vi "Spy Flush and Check for Specific Call.vi"(8 "error in (no error)":errorcluster, 10 "Specific Call":string, 11 "Mock Rig Process In":refnum<class "Mock Process.lvclass">) -> (0 "error out":errorcluster, 2 "Occured?":bool, 3 "Mock Rig Process Out":refnum<class "Mock Process.lvclass">)   [LabVIEW 2020, in "Mock Process.lvclass"]
uses:
  Mock Process.lvclass
  Mock Process.lvclass/Mock Process.ctl
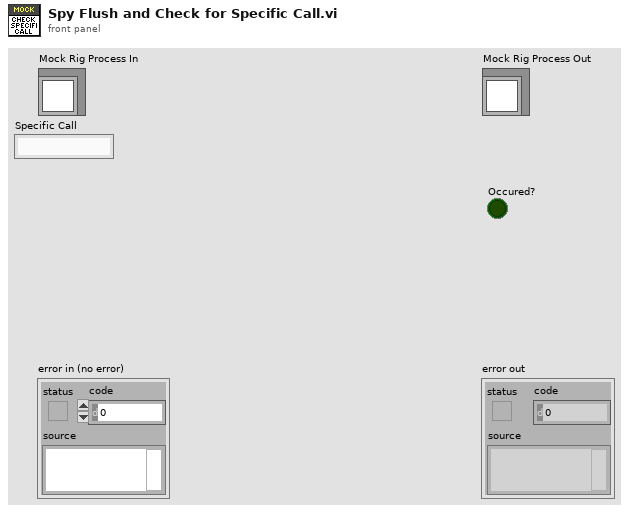
[diagram p1: front panel]
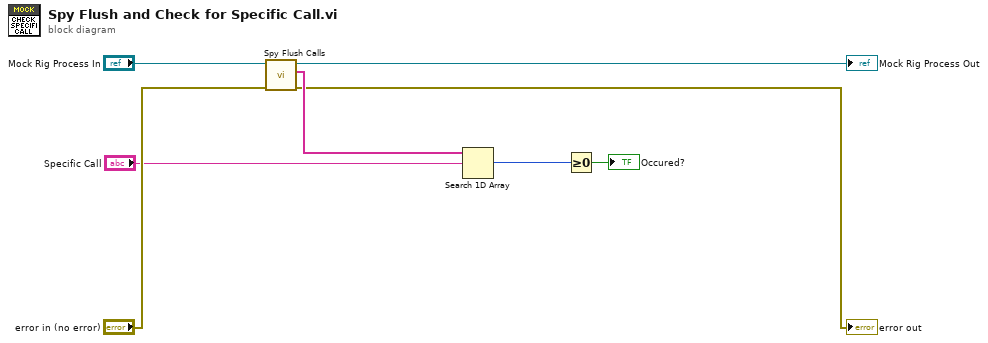
[diagram p0: block diagram]
diagram:
  n1 = call "Spy Flush Calls.vi"("error in (no error)"="error in (no error)", "Mock Process In"="Mock Rig Process In") -> ("error out"=→"error out":errorcluster, "Message"=w5:string[], "Mock Process Out"=→"Mock Rig Process Out":refnum<class "Mock Process.lvclass">)  [unwired: 6 in, 1 out]
  n2 = Search 1D Array(1D array=w5, element="Specific Call") -> (index of element=w3:i32)  [unwired: 1 in]
  n3 = Greater Or Equal To 0?(x=w3) -> (x >= 0?=→"Occured?":bool)
